vi "Configure Sequence (Trapezoid).vi"(0 "VISA resource name":refnum<visa-resource-name>, 1 "Channel Name (1)":string="1", 3 "Trapezoid Sequence Rise Time (1.0 s)":dbl=1.0 format="%^.3e", 4 "Waveform Type (1: Voltage)":i32(ring)=1 items=["Voltage"=1, "Current"=0], 5 "error in (no error)":errorcluster {"code" format="%.0x"}, 6 "Trapezoid Sequence Start Time (0.0 s)":dbl format="%^.3e", 7 "Trapezoid Sequence End Time (0.0 s)":dbl format="%^.3e", 8 "Trapezoid Sequence Start Level (0.0)":dbl format="%^.3e", 9 "Trapezoid Sequence Peak (0.0)":dbl format="%^.3e", 10 "Trapezoid Sequence Peak Width (1.0 s)":dbl=1.0 format="%^.3e", 11 "Trapezoid Sequence Fall Time (1.0 s)":dbl=1.0 format="%^.3e", 12 "Sequence Step Number (0)":i32) -> (14 "VISA resource name out":refnum<visa-resource-name>, 19 "error out":errorcluster {"code" format="%.0x"})   [LabVIEW 2016, in "Agilent N6700 Series.lvlib"]
doc: "Configures the trapezoid sequence.\n\n<b>Note:</b>\nThis VI only applies to the N6705B and N6705C DC Power Analyzer."
uses:
  <instrlib>/Agilent N6700 Series/Agilent N6700 Series.lvlib
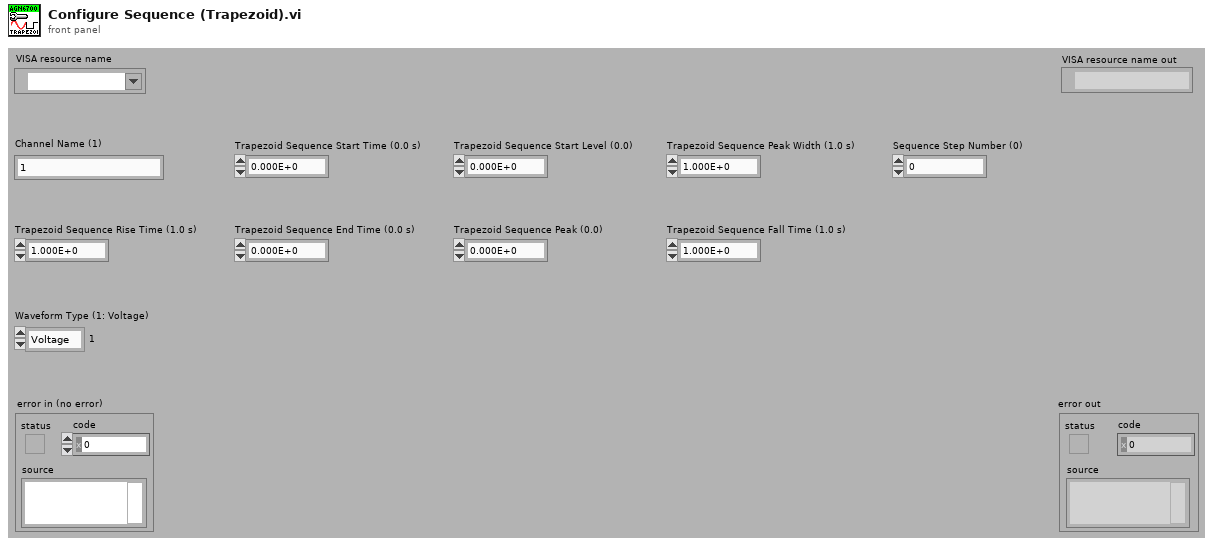
[diagram p1: front panel]
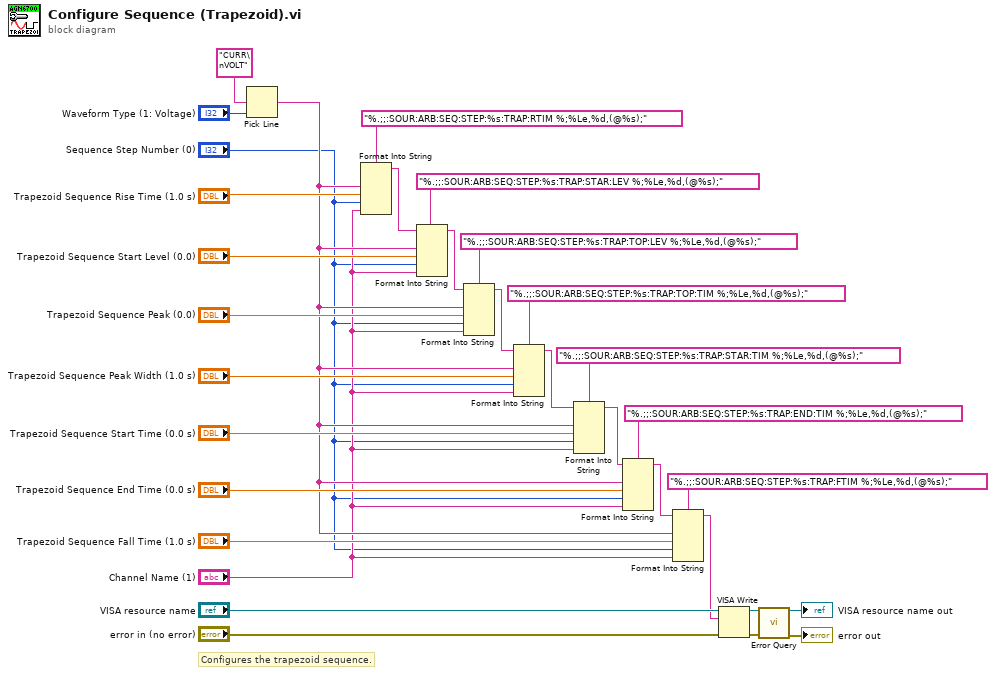
[diagram p0: block diagram]
diagram:
  # "Configures the trapezoid sequence."
  n1 = Pick Line(multi-line string="CURR\nVOLT", line index="Waveform Type (1: Voltage)") -> (output string=w3:string)  [unwired: 1 in]
  n2 = Format Into String(format string="%.;;:SOUR:ARB:SEQ:STEP:%s:TRAP:RTIM %;%Le,%d,(@%s);", w3, "Trapezoid Sequence Rise Time (1.0 s)", "Sequence Step Number (0)", "Channel Name (1)") -> (resulting string=w4:string)  [unwired: 2 in, 1 out]
  n3 = Format Into String(format string="%.;;:SOUR:ARB:SEQ:STEP:%s:TRAP:STAR:LEV %;%Le,%d,(@%s);", initial string=w4, w3, "Trapezoid Sequence Start Level (0.0)", "Sequence Step Number (0)", "Channel Name (1)") -> (resulting string=w22:string)  [unwired: 1 in, 1 out]
  n4 = Format Into String(format string="%.;;:SOUR:ARB:SEQ:STEP:%s:TRAP:TOP:LEV %;%Le,%d,(@%s);", initial string=w22, w3, "Trapezoid Sequence Peak (0.0)", "Sequence Step Number (0)", "Channel Name (1)") -> (resulting string=w21:string)  [unwired: 1 in, 1 out]
  n5 = Format Into String(format string="%.;;:SOUR:ARB:SEQ:STEP:%s:TRAP:TOP:TIM %;%Le,%d,(@%s);", initial string=w21, w3, "Trapezoid Sequence Peak Width (1.0 s)", "Sequence Step Number (0)", "Channel Name (1)") -> (resulting string=w20:string)  [unwired: 1 in, 1 out]
  n6 = Format Into String(format string="%.;;:SOUR:ARB:SEQ:STEP:%s:TRAP:STAR:TIM %;%Le,%d,(@%s);", initial string=w20, w3, "Trapezoid Sequence Start Time (0.0 s)", "Sequence Step Number (0)", "Channel Name (1)") -> (resulting string=w19:string)  [unwired: 1 in, 1 out]
  n7 = Format Into String(format string="%.;;:SOUR:ARB:SEQ:STEP:%s:TRAP:END:TIM %;%Le,%d,(@%s);", initial string=w19, w3, "Trapezoid Sequence End Time (0.0 s)", "Sequence Step Number (0)", "Channel Name (1)") -> (resulting string=w11:string)  [unwired: 1 in, 1 out]
  n8 = Format Into String(format string="%.;;:SOUR:ARB:SEQ:STEP:%s:TRAP:FTIM %;%Le,%d,(@%s);", initial string=w11, w3, "Trapezoid Sequence Fall Time (1.0 s)", "Sequence Step Number (0)", "Channel Name (1)") -> (resulting string=w9:string)  [unwired: 1 in, 1 out]
  n9 = VISA Write(VISA resource name="VISA resource name", write buffer=w9, error in (no error)="error in (no error)") -> (VISA resource name out=w28:refnum<visa-resource-name>, error out=w27:errorcluster)  [unwired: 1 out]
  n10 = call <instrlib>:"Error Query.vi"("VISA resource name"=w28, "error in (no error)"=w27) -> ("VISA resource name out"=→"VISA resource name out":refnum<visa-resource-name>, "error out"=→"error out":errorcluster)  [unwired: 10 in, 2 out]
